vi "distance.vi"(1 "read buffer":string) -> (0 "输出簇":cluster{"前距离\n":u16, "后距离":u16})   [LabVIEW 2014]
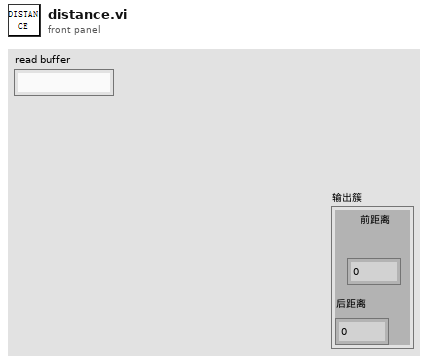
[diagram p1: front panel]
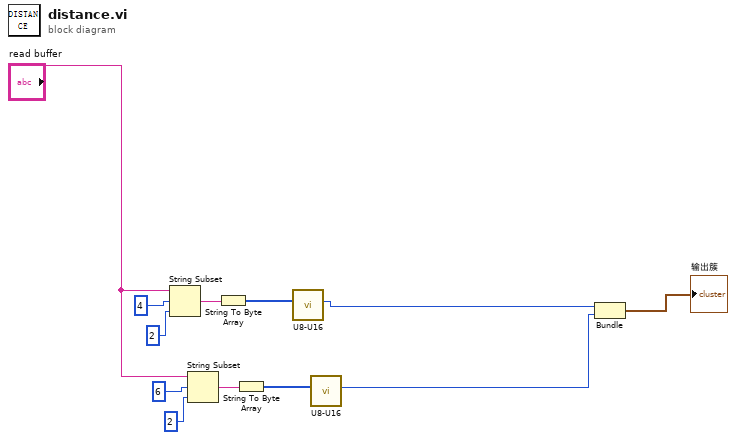
[diagram p0: block diagram]
diagram:
  n1 = String Subset(string="read buffer", offset (0)=4 ("长度（剩余）"), length (rest)=2 ("长度（剩余）")) -> (substring=w12:string)
  n2 = String Subset(string="read buffer", offset (0)=6 ("长度（剩余）"), length (rest)=2 ("长度（剩余）")) -> (substring=w6:string)
  n3 = String To Byte Array(string=w12) -> (unsigned byte array=w8:u8[])
  n4 = String To Byte Array(string=w6) -> (unsigned byte array=w3:u8[])
  n5 = call "U8-U16.vi"("数组"=w8) -> ("16位整型"=w7:u16)  [unwired: 8 in, 1 out]
  n6 = call "U8-U16.vi"("数组"=w3) -> ("16位整型"=w1:u16)  [unwired: 8 in, 1 out]
  n7 = Bundle("16位整型"=w7, "16位整型"=w1) -> (→"输出簇":cluster{"16位整型":u16, "16位整型":u16})  [unwired: 1 in]
